vi "数据查询_仪器日志.vi"() -> ()   [LabVIEW 2016, in "数据查询.lvlib"]
uses:
  <vilib>/Utility/miscctls.llb/LVPointTypeDef.ctl
  <vilib>/Utility/miscctls.llb/LVRowAndColumnUnsignedTypeDef.ctl
  <userlib>/_LVST/sqlite_api/Core/Select/SQLite_Select Str.vi
  <userlib>/_OpenG.lib/array/array.llb/Sort 2D Array (String)__ogtk.vi
  <userlib>/_LVST/sqlite_api/Core/Tables/SQLite_List Columns.vi
  <vilib>/addons/database/_DB Variant To Data/Database Variant To Data.xnode
panel:
  in  "列表框":i32(listbox)
  in  "页":i32 format="第%.0f页"
  in  "每页条数":i32=1000
  in  "向后按钮":bool
  in  "向前按钮":bool
  in  "导出":bool
  in  "查询":bool
  out "数据表":string[][](table)
  in  "结束日期":string="2050/01/01"
  in  "起始日期":string="2010/01/01"
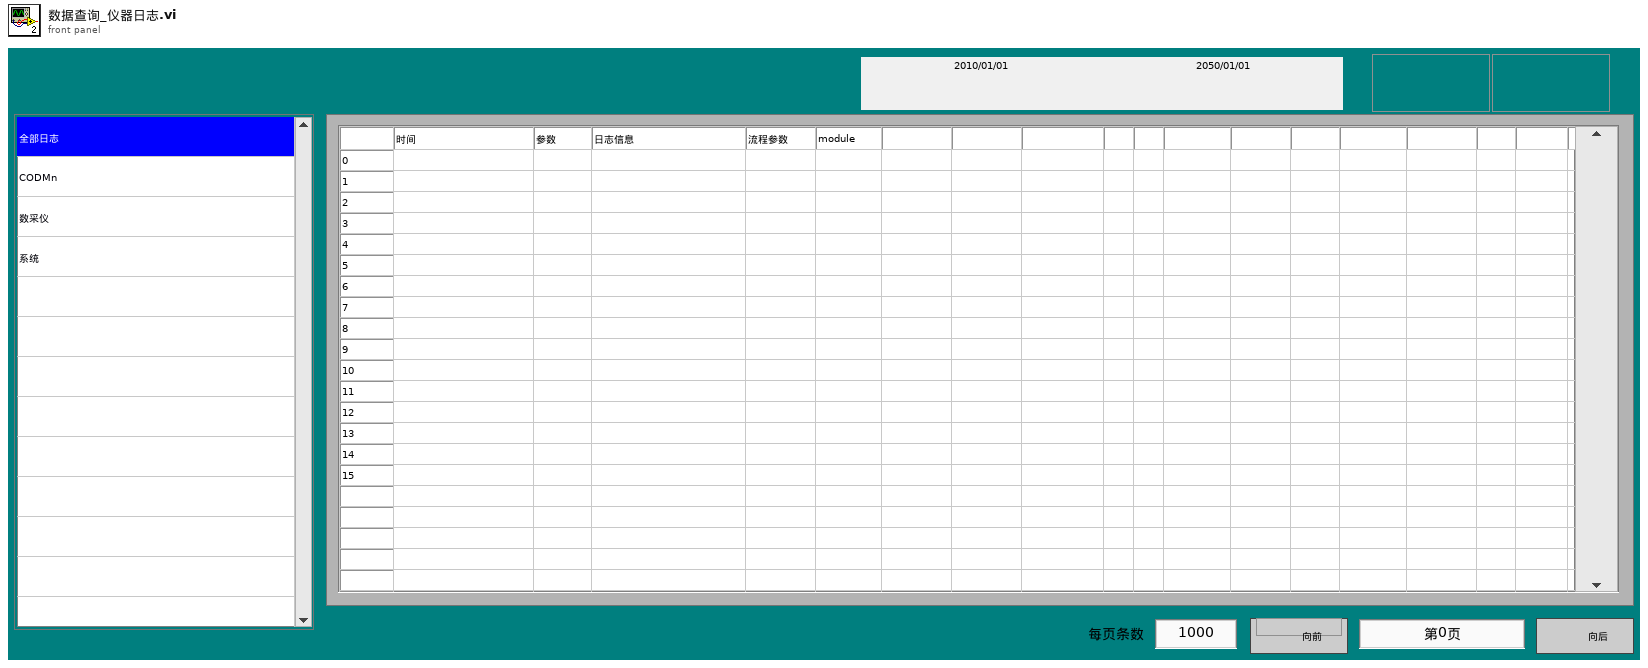
[diagram p1: front panel]
types:
  T1 = typedef "LVPointTypeDef.ctl" = cluster{"Horizontal":i16, "Vertical":i16}
  T2 = typedef "LVDateTimeRec.ctl" = cluster{"秒数的小数部分":dbl, "秒":i32, "分":i32, "时":i32, "日":i32, "月":i32, "年":i32, "天数（周）":i32, "天数（年）":i32, "DST":i32}
  T3 = typedef "数据查询菜单.xctl/数据 1.ctl" = enum32{"数据查询", "仪器数据", "仪器日志", "报警信息", "校准日志"}
  T4 = enum8{"Enabled", "Disabled", "Disabled and Grayed Out"}
  T5 = typedef "LVRowAndColumnUnsignedTypeDef.ctl" = cluster{"Row":u32, "Column":u32}
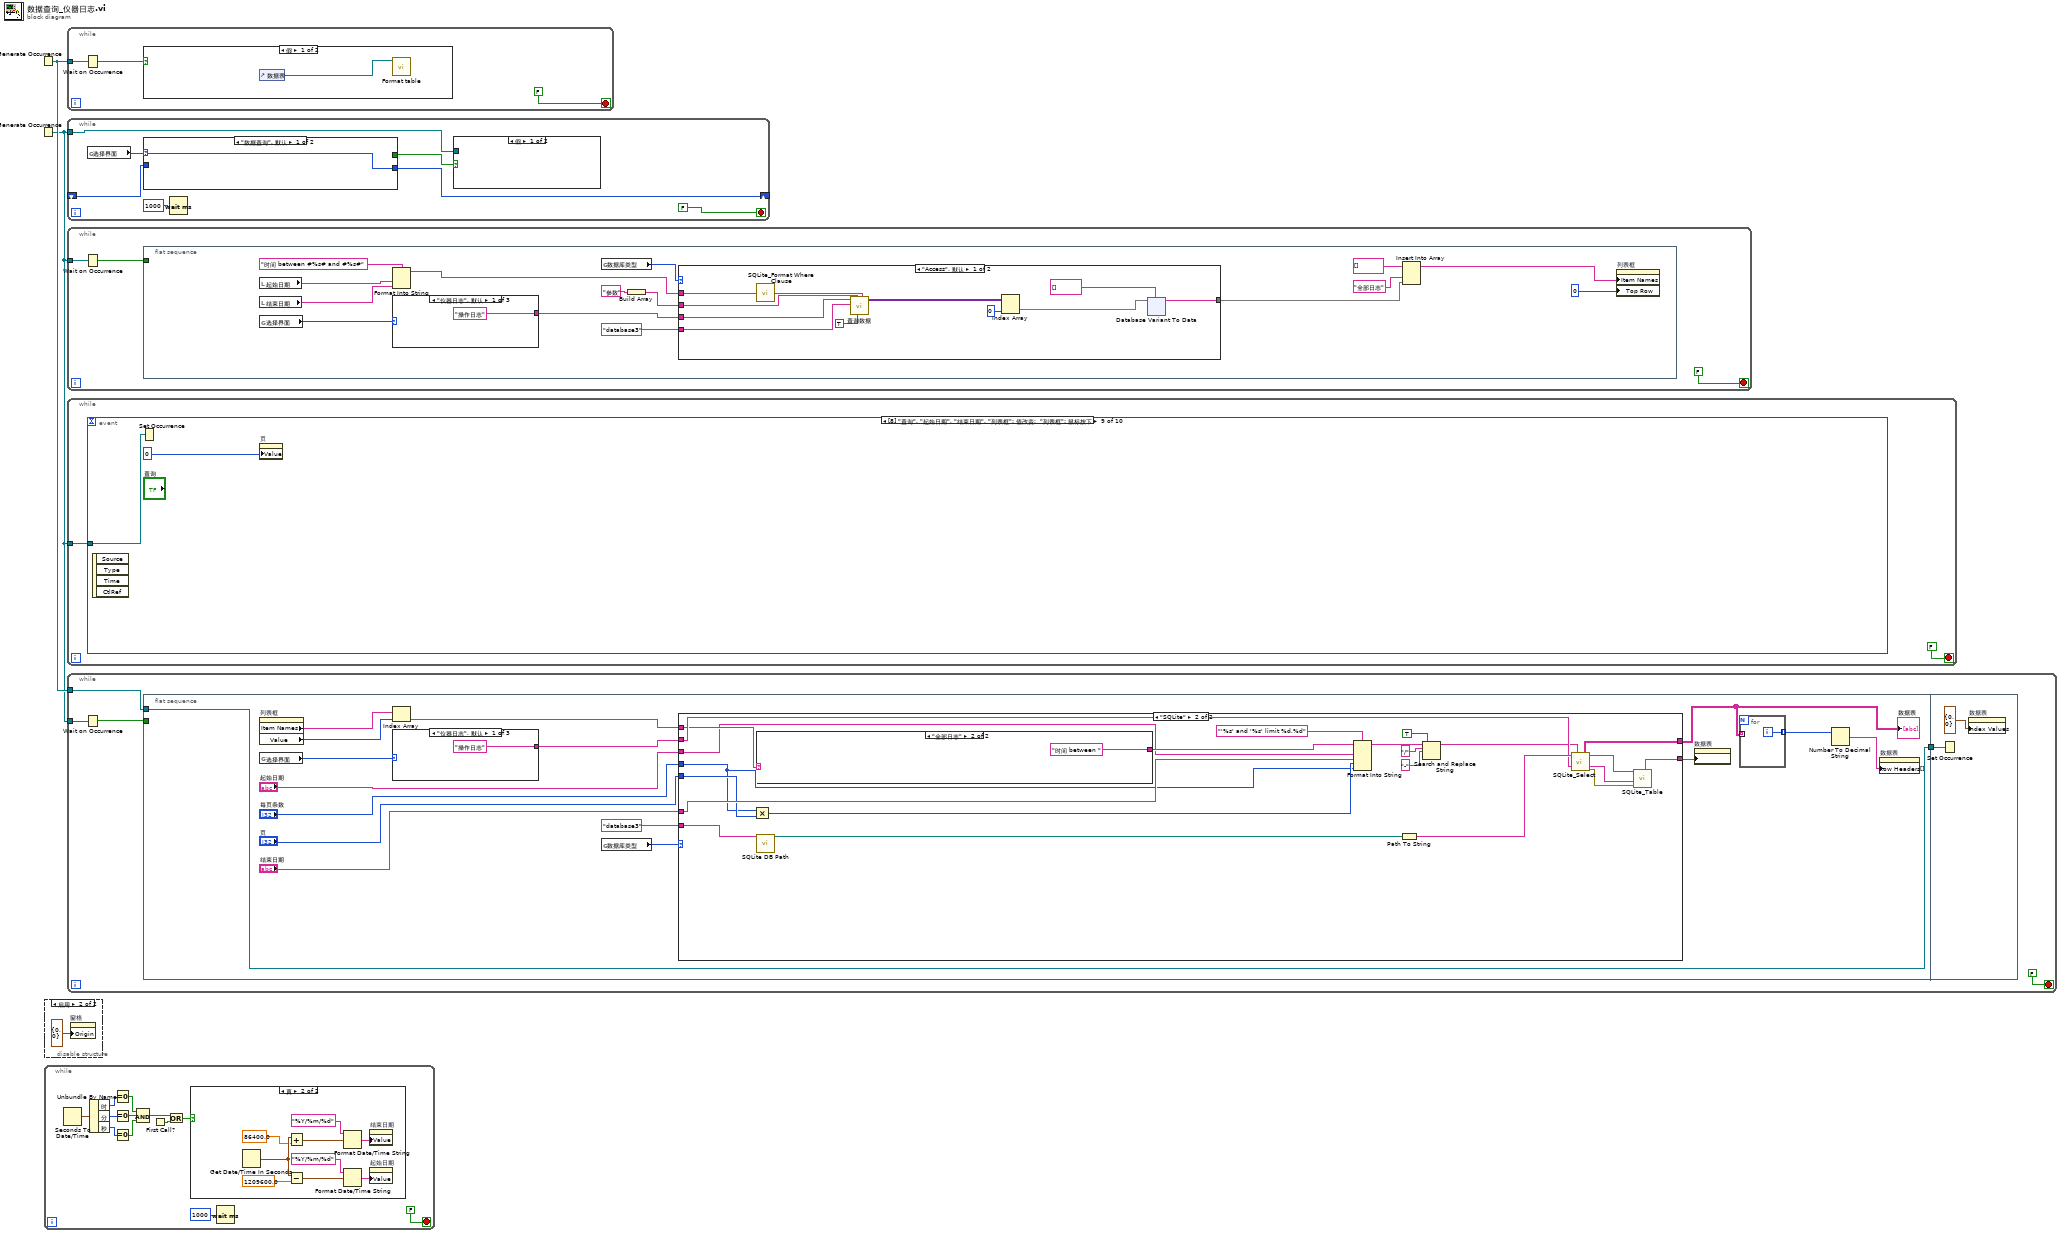
[diagram p0: block diagram]
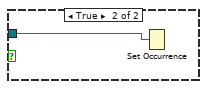
[diagram p2: hidden frame]
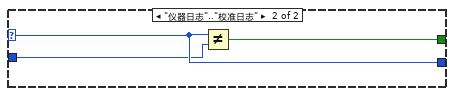
[diagram p3: hidden frame]
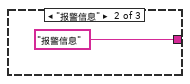
[diagram p5: hidden frame]
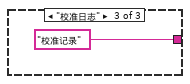
[diagram p6: hidden frame]
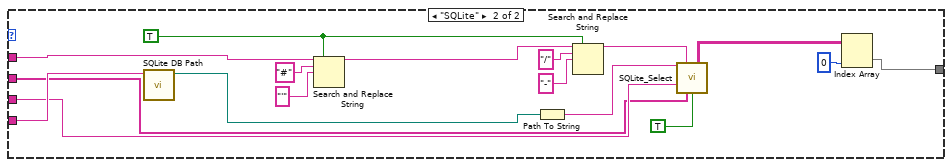
[diagram p7: hidden frame]
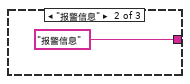
[diagram p8: hidden frame]
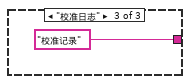
[diagram p9: hidden frame]
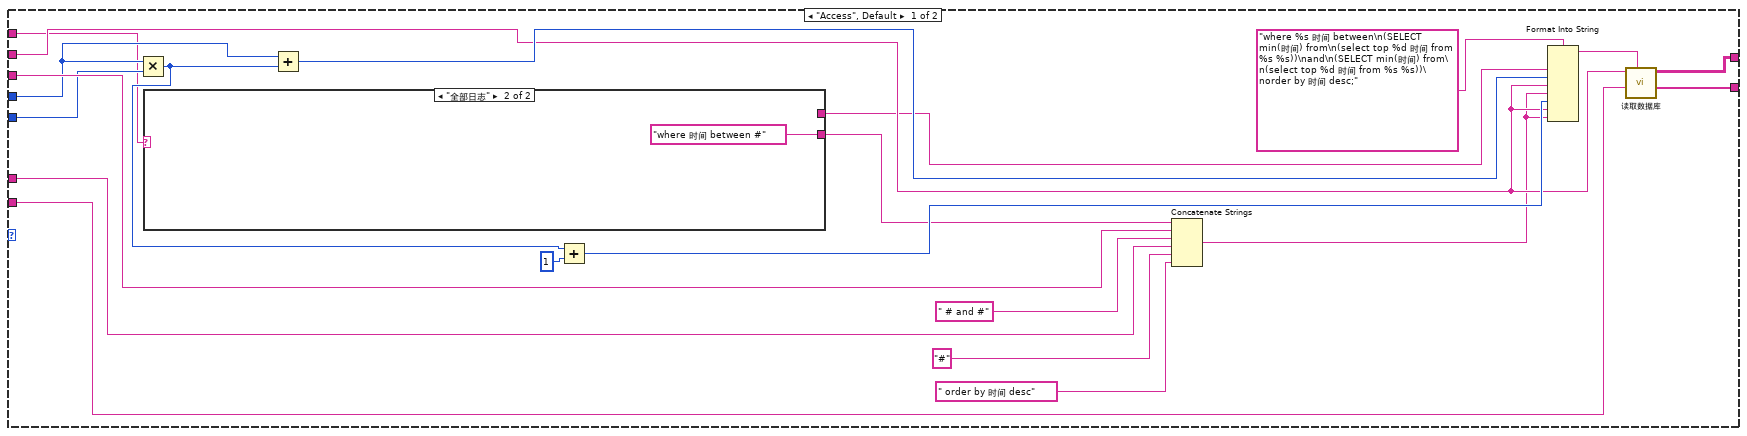
[diagram p10: hidden frame]
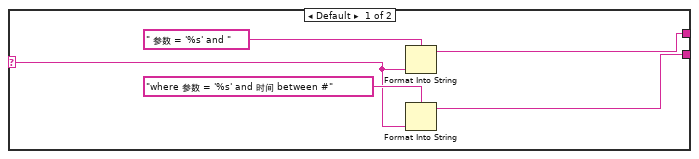
[diagram p11: hidden frame]
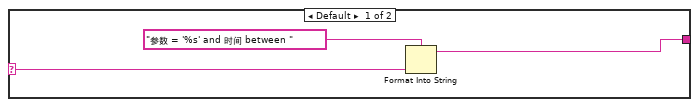
[diagram p12: hidden frame]
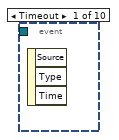
[diagram p14: hidden frame]
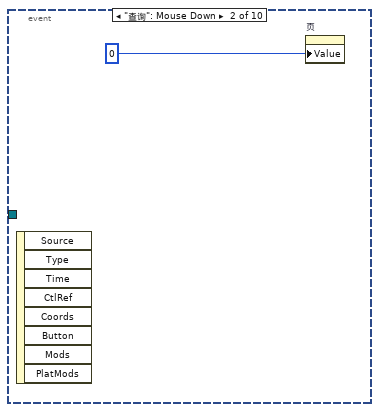
[diagram p15: hidden frame]
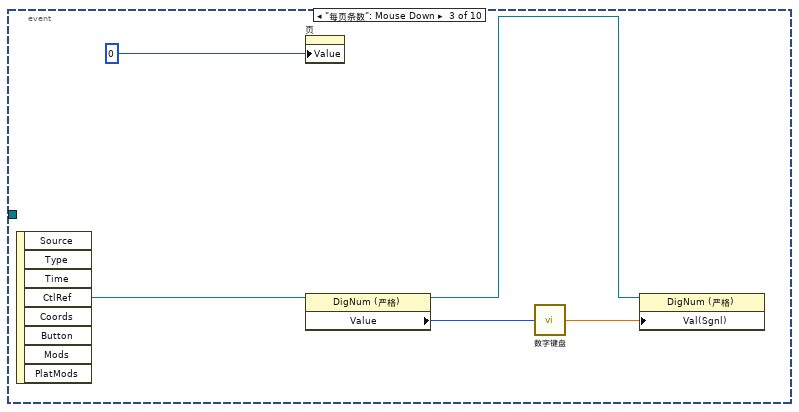
[diagram p16: hidden frame]
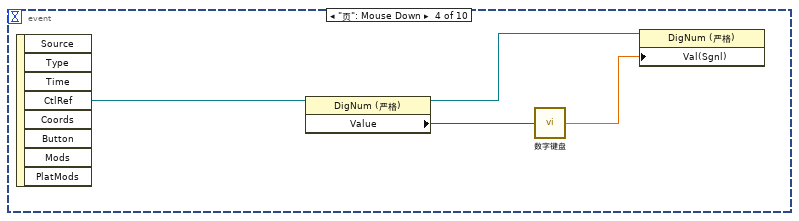
[diagram p17: hidden frame]
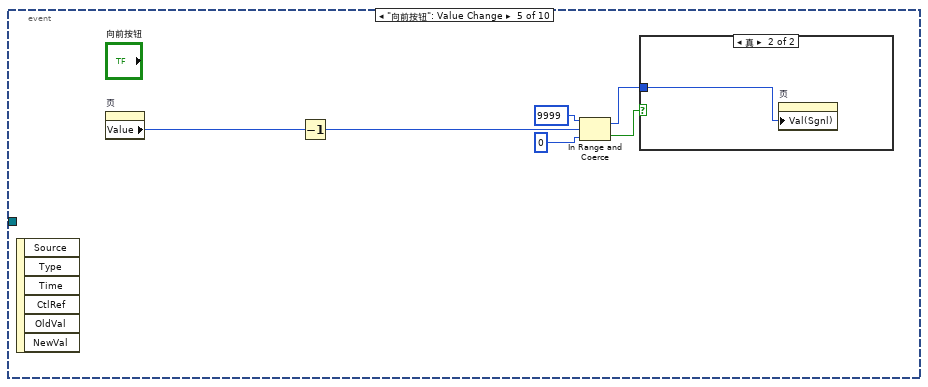
[diagram p18: hidden frame]
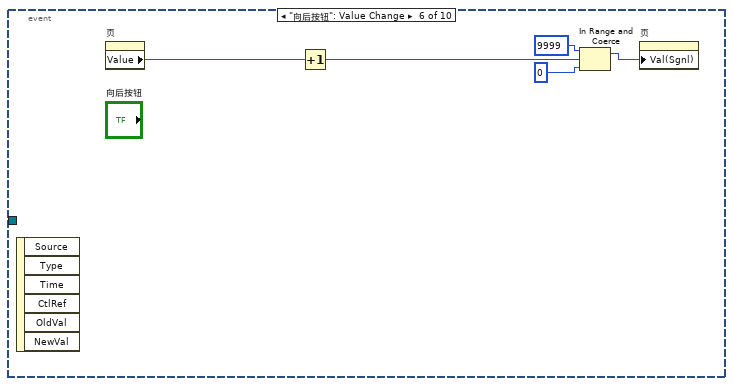
[diagram p20: hidden frame]
diagram:
  n1 = Generate Occurrence() -> (w2:refnum<k4>)
  n2 = Generate Occurrence() -> (w1:refnum<k4>)
  n3 = disable-structure shown="启用" {
    frame Disabled {
    }
    frame Enabled {
      n4 = property on="窗格" class="Pane"("Origin"=T1 {"Horizontal"=0, "Vertical"=0} ("原点")) -> ()  [unwired: 2 in, 2 out]
    }
  }
  n5 = while {
    stop <- FALSE stop-if-true
    n6 = Seconds To Date/Time() -> (date time rec=w15:T2)  [unwired: 2 in]
    n7 = Unbundle By Name(w15) -> ("时"=w14:i32, "分"=w13:i32, "秒"=w12:i32)
    n8 = Equal To 0?(x=w14) -> (x = 0?=w11:bool)
    n9 = Equal To 0?(x=w13) -> (x = 0?=w10:bool)
    n10 = Equal To 0?(x=w12) -> (x = 0?=w9:bool)
    n11 = Compound Arithmetic op=AND ("复合运算")(w11, w10, w9) -> (w6:bool)
    n12 = First Call?() -> (First Call?: T/F=w5:bool)
    n13 = Or(x=w6, y=w5) -> (x .or. y?=w4:bool)
    n14 = case shown="真" w4 {
      frame False {
      }
      frame True {
        n15 = Get Date/Time In Seconds() -> (seconds since 1Jan1904=w20:timestamp)
        n16 = Add(x=w20, y=86400.0) -> (x+y=w18:timestamp)
        n17 = Subtract(x=w20, y=1209600.0) -> (x-y=w21:timestamp)
        n18 = Format Date/Time String(time format string (%c)="%Y/%m/%d" ("时间格式字符串(%c)"), seconds (now)=w18) -> (date/time string=w17:string)  [unwired: 1 in]
        n19 = Format Date/Time String(time format string (%c)="%Y/%m/%d" ("时间格式字符串(%c)"), seconds (now)=w21) -> (date/time string=w23:string)  [unwired: 1 in]
        n20 = property on="结束日期" class="Str"("Value"=w17) -> ()  [unwired: 2 in, 2 out]
        n21 = property on="起始日期" class="Str"("Value"=w23) -> ()  [unwired: 2 in, 2 out]
      }
    }
    n22 = Wait (ms)(milliseconds to wait=u32 1000 ("等待时间（毫秒）")) -> ()  [unwired: 1 out]
  }
  n23 = while {
    tunnel: w2 -> [w25]
    stop <- FALSE stop-if-true
    n24 = Wait on Occurrence(2:w25) -> (0:w27:bool)  [unwired: 2 in]
    n25 = case shown="假" w27 {
      frame False {
        n26 = control-ref of="数据表"() -> (w28:refnum<vi>)
        n27 = call "Format table.vi"("Table输入"=w28) -> ()  [unwired: 11 in]
      }
      frame True {
      }
    }
  }
  n28 = while {
    shift-right: [w32] -> _
    shift-left: _ -> [w31]
    tunnel: w1 -> [w29]
    stop <- FALSE stop-if-true
    n29 = global read "全局变量.vi" "选择界面"() -> (w33:T3)
    n30 = case shown="\"数据查询\", 默认" w33 {
      selector: w33 -> [w37 w40]
      tunnel: [w37 w40] -> w32
      tunnel: w31 -> [_ w39]
      tunnel: [_ w38] -> w30
      frame "数据查询", Default {
      }
      frame "仪器日志".."校准日志" {
        n31 = Not Equal?(x=w40, y=w39) -> (x != y?=w38:bool)
      }
    }
    n32 = Wait (ms)(milliseconds to wait=u32 1000 ("等待时间（毫秒）")) -> ()  [unwired: 1 out]
    n33 = case shown="假" w30 {
      tunnel: w29 -> [_ w36]
      frame False {
      }
      frame True {
        n34 = Set Occurrence(w36) -> ()
      }
    }
  }
  n35 = while {
    tunnel: w1 -> [w41]
    stop <- FALSE stop-if-true
    n36 = Wait on Occurrence(2:w41) -> (0:w42:bool)  [unwired: 2 in]
    n37 = flat-sequence {
      tunnel: w42 -> [_]
      frame #0 {
        n38 = local read "起始日期"() -> (w54:string)
        n39 = local read "结束日期"() -> (w53:string)
        n40 = global read "全局变量.vi" "选择界面"() -> (w45:T3)
        n41 = Format Into String(format string="时间 between #%s# and #%s#" ("格式字符串"), w54, w53) -> (resulting string=w49:string)  [unwired: 2 in, 1 out]
        n42 = case shown="\"仪器日志\", 默认" w45 {
          tunnel: ["操作日志" "报警信息" "校准记录"] -> w44
          frame "仪器日志", Default {
          }
          frame "报警信息" {
          }
          frame "校准日志" {
          }
        }
        n43 = global read "全局变量.vi" "数据库类型"() -> (w46:enum16{"Access", "SQLite"})
        n44 = Build Array("参数") -> (w48:string[])
        n45 = case shown="\"Access\", 默认" w46 {
          tunnel: w44 -> [w72 w124]
          tunnel: w48 -> [w71 w123]
          tunnel: [w65 w119] -> w50
          tunnel: w49 -> [w64 w118]
          tunnel: "database3" ("database") -> [w62 w127]
          frame "Access", Default {
            n46 = call <userlib>:"SQLite_Format Where Clause.vi"("Where clause"=w64) -> ("String"=w63:string)  [unwired: 4 in]
            n47 = call "查询数据.vi"("condition"=w63, "Distinct"=TRUE, "columns"=w71, "database"=w62, "table"=w72) -> ("data"=w70:variant[][])  [unwired: 5 in, 1 out]
            n48 = Index Array(array=w70, index (col)=0 ("禁用的索引 (列)")) -> (element=w69:variant[])  [unwired: 1 in]
            n49 = xnode "Database Variant To Data"("database variant"=w69, "type"=string[] []) -> ("data"=w65:string[])  [unwired: 1 in, 1 out]
          }
          frame "SQLite" {
            w111 = TRUE ("替换全部？(F)")
            n50 = call "SQLite DB Path.vi"("database"=w127) -> ("appended path"=w126:path)  [unwired: 10 in]
            n51 = Search and Replace String(replace all?=w111, input string=w118, search string="#" ("搜索字符串"), replace string="'" ("替换字符串(\"\")")) -> (result string=w113:string)  [unwired: 4 in, 3 out]
            n52 = Path To String(path=w126) -> (string=w125:string)
            n53 = Search and Replace String(replace all?=w111, input string=w113, search string="/" ("搜索字符串"), replace string="-" ("替换字符串(\"\")")) -> (result string=w112:string)  [unwired: 4 in, 3 out]
            n54 = call-poly <userlib>:"SQLite_Select.vi"("DB Path"=w125, "Where Clause"=w112, "Table Name"=w124, "Columns"=w123, "Distinct"=TRUE) -> ("Results"=w121:string[][])  [unwired: 7 in, 3 out]
            n55 = Index Array(array=w121, index (col)=0 ("禁用的索引 (列)")) -> (element=w119:string[])  [unwired: 1 in]
          }
        }
        n56 = Insert Into Array(array=string[] [], new element #1="全部日志" ("新元素/子数组"), new element #2=w50) -> (w52:string[])  [unwired: 1 in]
        n57 = property on="列表框" class="LstBox (严格)"("Item Names"=w52, "Top Row"=0 ("顶行")) -> ()  [unwired: 2 in, 2 out]
      }
    }
  }
  n58 = while {
    tunnel: w1 -> [w128]
    stop <- FALSE stop-if-true
    n59 = event shown="[8] \"查询\", \"起始日期\", \"结束日期\", \"列表框\": 值改变;  \"列表框\": 鼠标按下" {
      selector: _ -> [_ _ _ _ _ _ _ _ _ _]
      dyn-events: _ -> [_ _ _ _ _ _ _ _ _ _]
      timeout: _ -> [_ _ _ _ _ _ _ _ _ _]
      tunnel: w128 -> [_ _ _ _ _ _ _ _ w197 w198]
      event Timeout {
        n60 = event-data() -> ()  [unwired: 1 in, 3 out]
      }
      event "查询": Mouse Down {
        n61 = event-data() -> ()  [unwired: 1 in, 8 out]
        n62 = property on="页" class="DigNum (严格)"("Value"=0 ("页")) -> ()  [unwired: 2 in, 2 out]
      }
      event "每页条数": Mouse Down {
        n63 = event-data() -> ("CtlRef"=w135:refnum<vi>)  [unwired: 1 in, 7 out]
        n64 = property on="页" class="DigNum (严格)"("Value"=0 ("页")) -> ()  [unwired: 2 in, 2 out]
        n65 = property class="DigNum (严格)"(reference=w135) -> (reference out=w132:refnum<vi>, "Value"=w134:i32)  [unwired: 1 in, 1 out]
        n66 = call "数字键盘.vi"("OldNumber"=w134) -> ("NewNumber"=w133:sgl)
        n67 = property class="DigNum (严格)"(reference=w132, "Val(Sgnl)"=w133) -> ()  [unwired: 1 in, 2 out]
      }
      event "页": Mouse Down {
        n68 = event-data() -> ("CtlRef"=w139:refnum<vi>)  [unwired: 1 in, 7 out]
        n69 = property class="DigNum (严格)"(reference=w139) -> (reference out=w136:refnum<vi>, "Value"=w138:i32)  [unwired: 1 in, 1 out]
        n70 = call "数字键盘.vi"("OldNumber"=w138) -> ("NewNumber"=w137:sgl)
        n71 = property class="DigNum (严格)"(reference=w136, "Val(Sgnl)"=w137) -> ()  [unwired: 1 in, 2 out]
      }
      event "向前按钮": Value Change {
        n72 = event-data() -> ()  [unwired: 1 in, 6 out]
        n73 = property on="页" class="DigNum (严格)"() -> ("Value"=w145:i32)  [unwired: 2 in, 2 out]
        n74 = Decrement(x=w145) -> (x-1=w144:i32)
        n75 = In Range and Coerce(upper limit=9999 ("上限"), x=w144, lower limit=0 ("下限")) -> (coerced(x)=w141:i32, In Range?=w140:bool)
        n76 = case shown="真" w140 {
          tunnel: w141 -> [_ w146]
          frame False {
          }
          frame True {
            n77 = property on="页" class="DigNum (严格)"("Val(Sgnl)"=w146) -> ()  [unwired: 2 in, 2 out]
          }
        }
      }
      event "向后按钮": Value Change {
        n78 = event-data() -> ()  [unwired: 1 in, 6 out]
        n79 = property on="页" class="DigNum (严格)"() -> ("Value"=w151:i32)  [unwired: 2 in, 2 out]
        n80 = Increment(x=w151) -> (x+1=w150:i32)
        n81 = In Range and Coerce(upper limit=u32 9999 ("上限"), x=w150, lower limit=u32 0 ("下限")) -> (coerced(x)=w147:u32)  [unwired: 1 out]
        n82 = property on="页" class="DigNum (严格)"("Val(Sgnl)"=w147) -> ()  [unwired: 2 in, 2 out]
      }
      event "导出": Value Change {
        n83 = event-data() -> ("CtlRef"=w152:refnum<vi>)  [unwired: 1 in, 5 out]
        n84 = property class="Bool"(reference=w152, "DisabledEnum"=T4."Disabled and Grayed Out" ("禁用")) -> (reference out=w156:refnum<vi>, error out=w157:errorcluster)  [unwired: 1 in]
        n85 = flat-sequence {
          tunnel: w157 -> [_]
          tunnel: [w176] -> w155
          tunnel: w156 -> [w176]
          tunnel: "导出" -> [_]
          frame #0 {
            n86 = property on="列表框" class="LstBox (严格)"() -> ("Item Names"=w161:string[], "Value"=w160:i32)  [unwired: 2 in, 2 out]
            n87 = property on="数据表" class="Tbl (严格)"() -> ("Column Headers[]"=w169:string[])  [unwired: 2 in, 2 out]
            n88 = local read "数据表"() -> (w180:string[][])
            n89 = Index Array(array=w161, index=w160) -> (element=w159:string)
            n90 = Format Date/Time String(time format string (%c)="%y_%m_%d" ("时间格式字符串(%c)")) -> (date/time string=w173:string)  [unwired: 2 in]
            n91 = call-poly <userlib>:"Sort Array__ogtk.vi"("Column/Row to Sort By"=u32 0, "Sort By in"=enum16{"row", "column"}."column", "Order"=enum16{"ascending", "descending"}."ascending", "Array in"=w180) -> ("Sorted Array out"=w162:string[][])  [unwired: 4 in, 3 out]
            n92 = Concatenate Strings(w159, "_" ("字符串"), w173) -> (w171:string)
            n93 = for {
              tunnel: w162 -> [w189] mode=indexing
              tunnel: [w188] -> w166 mode=indexing
              i -> [w190]
              n94 = Increment(x=w190) -> (x+1=w186:i32)
              n95 = Number To Decimal String(number=w186) -> (decimal integer string=w185:string)  [unwired: 1 in]
              n96 = Insert Into Array(array=w189, index=0 ("索引"), new element=w185) -> (w188:string[])
            }
            n97 = Insert Into Array(array=w169, index=0 ("索引"), new element="序号" ("新元素/子数组")) -> (w170:string[])
            n98 = Insert Into Array(array=string[][] [], new element #1=w170, new element #2=w166) -> (w165:string[][])  [unwired: 2 in]
            n99 = call "数据导出Excel.vi"("text data"=w165, "default name"=w171) -> ("error out"=w164:errorcluster, "布尔"=w163:bool)  [unwired: 8 in]
            n100 = case shown="真" w163 {
              tunnel: w164 -> [_ w182]
              frame False {
              }
              frame True {
                n101 = case shown="错误" w182 {
                  tunnel: ["导出成功" ("消息") "导出失败" ("消息")] -> w181
                  frame No Error {
                  }
                  frame Error {
                  }
                }
                n102 = One Button Dialog(message=w181) -> ()  [unwired: 1 in, 1 out]
              }
            }
          }
        }
        n103 = property class="Bool"(reference=w155, "DisabledEnum"=T4."Enabled" ("禁用")) -> ()  [unwired: 1 in, 2 out]
      }
      event "起始日期", "结束日期": Mouse Down {
        n104 = event-data() -> ("CtlRef"=w195:refnum<vi>)  [unwired: 1 in, 7 out]
        n105 = property on="页" class="DigNum (严格)"("Value"=0 ("页")) -> ()  [unwired: 2 in, 2 out]
        n106 = property class="Str"(reference=w195) -> (reference out=w193:refnum<vi>, "Value"=w194:string)  [unwired: 1 in, 1 out]
        n107 = call "日期键盘.vi"("原值"=w194) -> ("x+y"=w192:string)  [unwired: 10 in]
        n108 = property class="Str"(reference=w193, "Val(Sgnl)"=w192) -> ()  [unwired: 1 in, 2 out]
      }
      event "查询", "起始日期", "结束日期", "列表框": Value Change; "列表框": Mouse Down {
        n109 = event-data() -> ()  [unwired: 1 in, 4 out]
        n110 = Set Occurrence(w197) -> ()
        n111 = property on="页" class="DigNum (严格)"("Value"=0 ("页")) -> ()  [unwired: 2 in, 2 out]
      }
      event "页", "每页条数": Value Change {
        n112 = event-data() -> ()  [unwired: 1 in, 6 out]
        n113 = Set Occurrence(w198) -> ()
      }
    }
  }
  n114 = while {
    tunnel: w1 -> [w202]
    tunnel: w2 -> [w199]
    stop <- FALSE stop-if-true
    n115 = Wait on Occurrence(2:w202) -> (0:w201:bool)  [unwired: 2 in]
    n116 = flat-sequence {
      tunnel: w201 -> [_]
      tunnel: [w215] -> w200
      tunnel: w199 -> [w215]
      tunnel: w200 -> [w277]
      frame #0 {
        n117 = property on="列表框" class="LstBox (严格)"() -> ("Item Names"=w216:string[], "Value"=w217:i32)  [unwired: 2 in, 2 out]
        n118 = global read "全局变量.vi" "选择界面"() -> (w205:T3)
        n119 = Index Array(array=w216, index=w217) -> (element=w212:string)
        n120 = case shown="\"仪器日志\", 默认" w205 {
          tunnel: ["操作日志" "报警信息" "校准记录"] -> w204
          frame "仪器日志", Default {
          }
          frame "报警信息" {
          }
          frame "校准日志" {
          }
        }
        n121 = global read "全局变量.vi" "数据库类型"() -> (w211:enum16{"Access", "SQLite"})
        n122 = case shown="\"SQLite\"" w211 {
          tunnel: "起始日期" -> [w243 w259]
          tunnel: "结束日期" -> [w242 w258]
          tunnel: [w239 w264] -> w214
          tunnel: [w237 w263] -> w213
          tunnel: "每页条数" -> [w231 w250]
          tunnel: "页" -> [w230 w252]
          tunnel: w204 -> [w229 w268]
          tunnel: "database3" ("database") -> [w227 w269]
          tunnel: w212 -> [w225 w262]
          frame "Access", Default {
            n123 = Multiply(x=w231, y=w230) -> (x*y=w235:i32)
            n124 = case shown="\"全部日志\"" w225 {
              selector: w225 -> [w245 _]
              tunnel: [w248 "where 时间 between #" ("condition")] -> w223
              tunnel: [w244 _] -> w224
              frame Default {
                n125 = Format Into String(format string=" 参数 = '%s' and " ("condition"), w245) -> (resulting string=w244:string)  [unwired: 2 in, 1 out]
                n126 = Format Into String(format string="where 参数 = '%s' and 时间 between #" ("condition"), w245) -> (resulting string=w248:string)  [unwired: 2 in, 1 out]
              }
              frame "全部日志" {
              }
            }
            n127 = Add(x=w231, y=w235) -> (x+y=w233:i32)
            n128 = Add(x=w235, y=u32 1) -> (x+y=w232:u32)
            n129 = Concatenate Strings(w223, w243, " # and #" ("condition"), w242, "#" ("condition"), " order by 时间 desc" ("字符串")) -> (w228:string)
            n130 = Format Into String(format string="where %s 时间 between\n(SELECT min(时间) from\n(select top %d 时间 from %s %s))\nand\n(SELECT min(时间) from\n(select top %d 时间 from %s %s))\norder by 时间 desc;" ("格式字符串"), w224, w233, w229, w228, w232, w229, w228) -> (resulting string=w226:string)  [unwired: 2 in, 1 out]
            n131 = call "读取数据库.vi"("condition"=w226, "database"=w227, "组合框"=w229) -> ("columns"=w239:string[], "表格"=w237:string[][])  [unwired: 5 in, 2 out]
          }
          frame "SQLite" {
            n132 = Multiply(x=w250, y=w252) -> (x*y=w251:i32)
            n133 = case shown="\"全部日志\"" w262 {
              selector: w262 -> [w272 _]
              tunnel: [w274 "时间 between " ("condition")] -> w261
              frame Default {
                n134 = Format Into String(format string="参数 = '%s' and 时间 between " ("condition"), w272) -> (resulting string=w274:string)  [unwired: 2 in, 1 out]
              }
              frame "全部日志" {
              }
            }
            n135 = call "SQLite DB Path.vi"("database"=w269) -> ("appended path"=w271:path)  [unwired: 10 in]
            n136 = Format Into String(format string="'%s' and '%s' limit %d,%d" ("格式字符串"), initial string=w261, w259, w258, w251, w250) -> (resulting string=w255:string)  [unwired: 1 in, 1 out]
            n137 = Path To String(path=w271) -> (string=w270:string)
            n138 = Search and Replace String(replace all?=TRUE ("替换全部？(F)"), input string=w255, search string="/" ("搜索字符串"), replace string="-" ("替换字符串(\"\")")) -> (result string=w254:string)  [unwired: 4 in, 3 out]
            n139 = call-poly <userlib>:"SQLite_Select.vi"("DB Path"=w270, "Where Clause"=w254, "Table Name"=w268) -> ("Results"=w263:string[][], "DB Path Out"=w267:string, "Table Name Out"=w266:string, "error out"=w265:errorcluster)  [unwired: 9 in]
            n140 = call-poly <userlib>:"SQLite_Table.vi"("DB Path"=w267, "Table Name"=w266, "error in (no error)"=w265) -> ("Columns"=w264:string[])  [unwired: 4 in, 3 out]
          }
        }
        "数据表" <- w213
        n141 = property on="数据表" class="Tbl (严格)"("Column Headers[]"=w214) -> ()  [unwired: 2 in, 2 out]
        n142 = for {
          tunnel: [w276] -> w219 mode=indexing
          tunnel: w213 -> [_] mode=indexing
          i -> [w276]
        }
        n143 = Number To Decimal String(number=w219) -> (decimal integer string=w218:string[])  [unwired: 1 in]
        n144 = property on="数据表" class="Tbl (严格)"("Row Headers[]"=w218) -> ()  [unwired: 2 in, 2 out]
      }
      frame #1 {
        n145 = Set Occurrence(w277) -> ()
        n146 = property on="数据表" class="Tbl (严格)"("Index Values"=T5 {"Row"=0, "Column"=0} ("索引值")) -> ()  [unwired: 2 in, 2 out]
      }
    }
  }
